vi "Delete Event.vi"(8 "error in (no error)":errorcluster, 10 "Name":string, 11 "State in":refnum<class "State.lvclass">) -> (0 "error out":errorcluster, 3 "State out":refnum<class "State.lvclass">)   [LabVIEW 2015, in "State.lvclass"]
uses:
  State.lvclass
  State.lvclass/State.ctl
  Termination/Termination.lvclass/Termination.ctl
  Termination/Read Source.vi
  Termination/Termination.lvclass
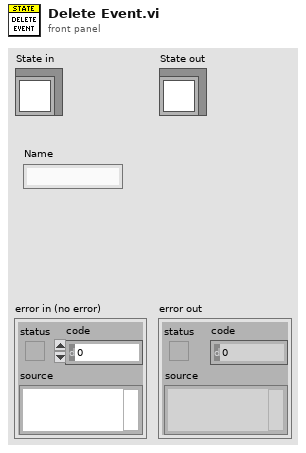
[diagram p1: front panel]
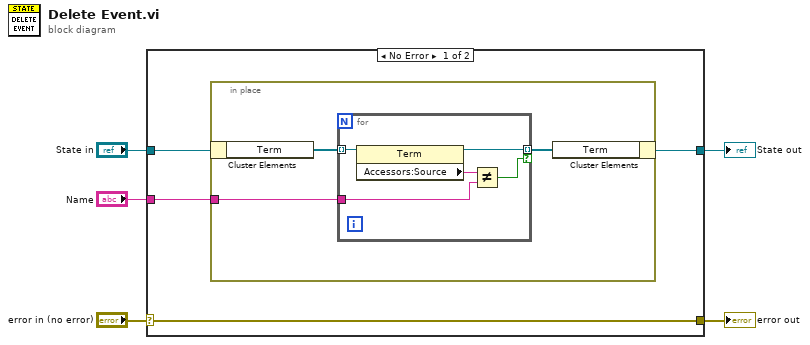
[diagram p0: block diagram]
diagram:
  n1 = case shown="No Error" "error in (no error)" {
    selector: "error in (no error)" -> [w9 w19]
    tunnel: [w9 w19] -> w4
    tunnel: [w7 w18] -> w2
    tunnel: "State in" -> [w8 w18]
    tunnel: "Name" -> [w6 _]
    frame No Error {
      n2 = in-place {
        in-place-border: w6 -> [w10]
        n3 = in-place-cluster #1(w8) -> ("Term"=w12:refnum<class "Termination.lvclass">[])
        n4 = for {
          tunnel: w12 -> [w17] mode=indexing
          tunnel: [w16] -> w11 mode=indexing if=w15
          tunnel: w10 -> [w13]
          n5 = property class="Term"(reference=w17) -> (reference out=w16:refnum<class "Termination.lvclass">, "Accessors:Source"=w14:string)  [unwired: 1 in, 1 out]
          n6 = Not Equal?(x=w14, y=w13) -> (x != y?=w15:bool)
        }
        n7 = in-place-cluster #1("Term"=w11) -> (w7:refnum<class "State.lvclass">)
      }
    }
    frame Error {
    }
  }
  "error out" <- w4
  "State out" <- w2
